vi "Physical Constants.vi"(1 "Input":dbl, 2 "Physical Constants FGV Selector":T1, 3 "Action":T2) -> (0 "Output":dbl)   [LabVIEW 2013]
uses:
  Action.ctl
  Physical Constants FGV Selector.ctl
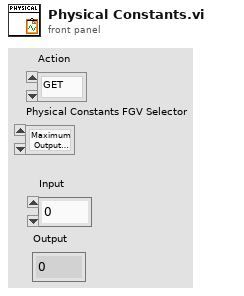
[diagram p1: front panel]
types:
  T1 = typedef "Physical Constants FGV Selector.ctl" = enum16{"Maximum Output Voltage", "Minimum Output Voltage", "Maximum Input Voltage", "Minimum Input Voltage"}
  T2 = typedef "Action.ctl" = enum16{"GET", "PUT", "DELETE"}
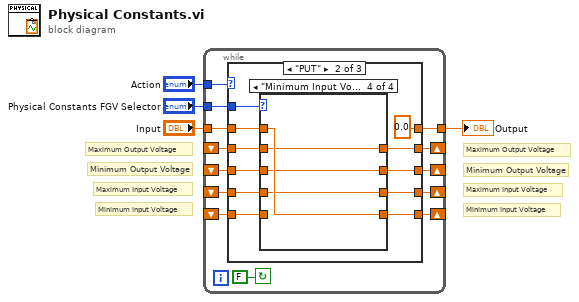
[diagram p0: block diagram]
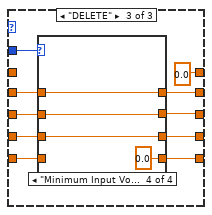
[diagram p9: hidden frame]
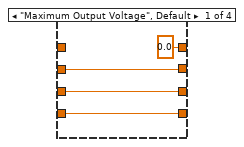
[diagram p10: hidden frame]
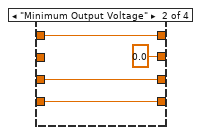
[diagram p11: hidden frame]
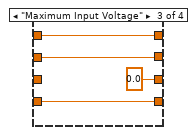
[diagram p12: hidden frame]
diagram:
  # "Minimum Input Voltage"
  # "Maximum Input Voltage"
  # "Minimum Output Voltage"
  # "Maximum Output Voltage"
  # "Minimum Input Voltage"
  # "Maximum Input Voltage"
  # "Minimum Output Voltage"
  # "Maximum Output Voltage"
  n1 = while {
    tunnel: "Action" -> [w16]
    tunnel: "Physical Constants FGV Selector" -> [w15]
    tunnel: "Input" -> [w14]
    tunnel: [w13] -> w2
    shift-right: [w11] -> _
    shift-left: _ -> [w12]
    shift-right: [w9] -> _
    shift-left: _ -> [w10]
    shift-right: [w7] -> _
    shift-left: _ -> [w8]
    shift-right: [w5] -> _
    shift-left: _ -> [w6]
    stop <- FALSE continue-if-true
    n2 = case shown="\"PUT\"" w16 {
      tunnel: w15 -> [w27 w53 w79]
      tunnel: w14 -> [_ w52 _]
      tunnel: [w18 0.0 0.0] -> w13
      tunnel: w12 -> [w25 w50 w74]
      tunnel: [w26 w51 w78] -> w11
      tunnel: w10 -> [w23 w48 w73]
      tunnel: [w24 w49 w77] -> w9
      tunnel: w8 -> [w21 w46 w72]
      tunnel: [w22 w47 w76] -> w7
      tunnel: w6 -> [w19 w44 w71]
      tunnel: [w20 w45 w75] -> w5
      frame "GET", Default {
        n3 = case shown="\"Minimum Input Voltage\"" w27 {
          tunnel: [w28 w35 w39 w43] -> w26
          tunnel: w25 -> [w28 w35 w39 w43]
          tunnel: [w31 w34 w38 w42] -> w24
          tunnel: w23 -> [w31 w34 w38 w42]
          tunnel: [w30 w33 w36 w41] -> w22
          tunnel: w21 -> [w30 w33 w36 w41]
          tunnel: [w29 w32 w37 w40] -> w20
          tunnel: w19 -> [w29 w32 w37 w40]
          tunnel: [w28 w34 w36 w40] -> w18
          frame "Maximum Output Voltage", Default {
          }
          frame "Minimum Output Voltage" {
          }
          frame "Maximum Input Voltage" {
          }
          frame "Minimum Input Voltage" {
          }
        }
      }
      frame "PUT" {
        n4 = case shown="\"Minimum Input Voltage\"" w53 {
          tunnel: w52 -> [w55 w62 w66 w70]
          tunnel: [w55 w61 w65 w67] -> w51
          tunnel: w50 -> [_ w61 w65 w67]
          tunnel: [w58 w62 w64 w68] -> w49
          tunnel: w48 -> [w58 _ w64 w68]
          tunnel: [w57 w60 w66 w69] -> w47
          tunnel: w46 -> [w57 w60 _ w69]
          tunnel: [w56 w59 w63 w70] -> w45
          tunnel: w44 -> [w56 w59 w63 _]
          frame "Maximum Output Voltage", Default {
          }
          frame "Minimum Output Voltage" {
          }
          frame "Maximum Input Voltage" {
          }
          frame "Minimum Input Voltage" {
          }
        }
      }
      frame "DELETE" {
        n5 = case shown="\"Minimum Input Voltage\"" w79 {
          tunnel: [0.0 w87 w91 w95] -> w78
          tunnel: [w81 0.0 w90 w94] -> w77
          tunnel: [w82 w86 0.0 w93] -> w76
          tunnel: [w83 w85 w89 0.0] -> w75
          tunnel: w74 -> [_ w87 w91 w95]
          tunnel: w73 -> [w81 _ w90 w94]
          tunnel: w72 -> [w82 w86 _ w93]
          tunnel: w71 -> [w83 w85 w89 _]
          frame "Maximum Output Voltage", Default {
          }
          frame "Minimum Output Voltage" {
          }
          frame "Maximum Input Voltage" {
          }
          frame "Minimum Input Voltage" {
          }
        }
      }
    }
  }
  "Output" <- w2
